vi "Write Module Configuration.vi"(8 "error in":errorcluster, 10 "module configuration":refnum<class "TBM module configuration.lvclass">, 11 "Module Editor Node in":refnum<class "module editor node.lvclass">) -> (0 "error out":errorcluster, 3 "Module Editor Node out":refnum<class "module editor node.lvclass">)   [LabVIEW 2013, in "PL Framework Configuration Tool.lvlib" / "module editor node.lvclass"]
uses:
  module editor node.lvclass
  <vilib>/NI/Tag Bus Module Framework/module configuration/TBM module configuration.lvclass
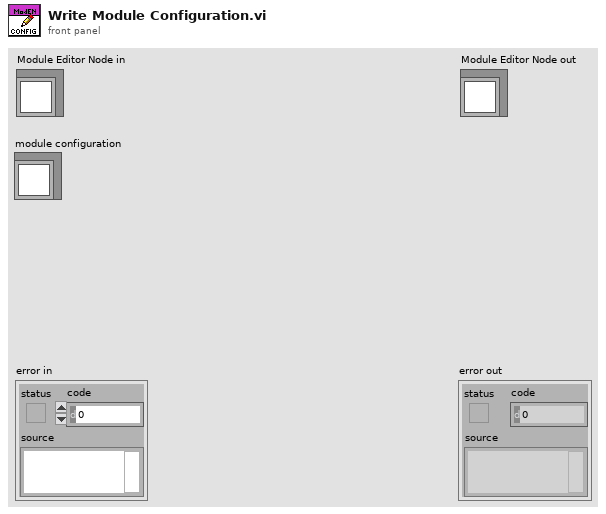
[diagram p1: front panel]
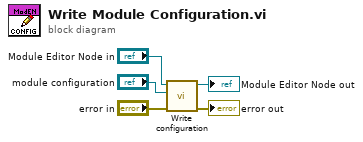
[diagram p0: block diagram]
diagram:
  n1 = call-dynamic "Write configuration.vi"("error in"="error in", "configuration"="module configuration", "NISE_CEF_serializable node in"="Module Editor Node in") -> ("error out"=→"error out":errorcluster, "NISE_CEF_serializable node out"=→"Module Editor Node out":refnum<class "module editor node.lvclass">)  [unwired: 7 in]
